vi "Get All Keys.vi"(8 "error in (no error)":errorcluster, 11 "Configuration In":refnum<class "Configuration.lvclass">) -> (0 "error out":errorcluster, 1 "Keys":string[](array[string]), 3 "Configuration Out":refnum<class "Configuration.lvclass">)   [LabVIEW 2020, in "Configuration.lvclass"]
doc: "High-level function for reading configuration file data from process class."
uses:
  Configuration.lvclass
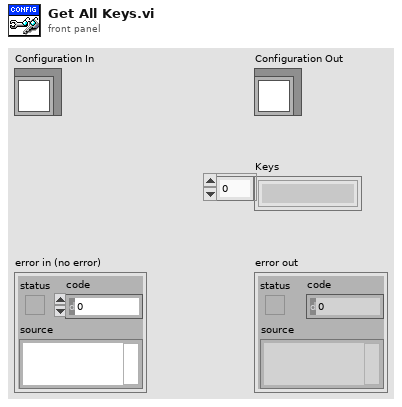
[diagram p1: front panel]
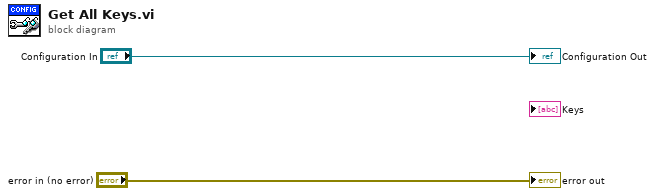
[diagram p0: block diagram]
diagram:
  "error out" <- "error in (no error)"
  "Configuration Out" <- "Configuration In"
